vi "build_config_trig (SubVI).vi"() -> (3 "config_trig":dbl[](array[numeric]))   [LabVIEW 2014]
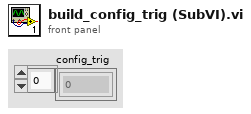
[diagram p1: front panel]
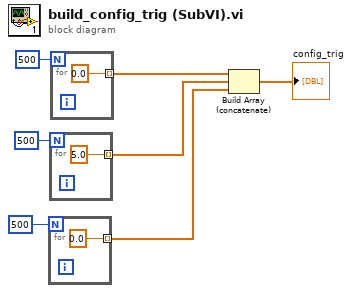
[diagram p0: block diagram]
diagram:
  n1 = for {
    N: 500 -> [_]
    tunnel: [0.0] -> w2 mode=indexing
  }
  n2 = for {
    N: 500 -> [_]
    tunnel: [5.0] -> w3 mode=indexing
  }
  n3 = for {
    N: 500 -> [_]
    tunnel: [0.0] -> w4 mode=indexing
  }
  n4 = Build Array (concatenate)(w4, w3, w2) -> (→"config_trig":dbl[])
